vi "optionsAcq_interferogramSmoothing.vi"(0 "reference":refnum<class "OSA200.lvclass">, 2 "smoothing":T1, 4 "readWrite":enum16{"read", "write"}(ring), 5 "error in (no error)":errorcluster, 6 "width":u16, 7 "ignore range violation (false)":bool, 8 "nrOfPasses":u16) -> (10 "nrOfPasses out":u16, 12 "width out":u16, 14 "duplicate reference":refnum<class "OSA200.lvclass">, 15 "status":string, 16 "smoothing out":T1, 19 "error out":errorcluster)   [LabVIEW 2010, in "OSA200.lvclass"]
uses:
  OSA200.lvclass
  _misc/Thorlabs_FTS_misc.llb/interferogram_smoothing.ctl
  OSA.lvclass
  OSA20X_misc.lvlib
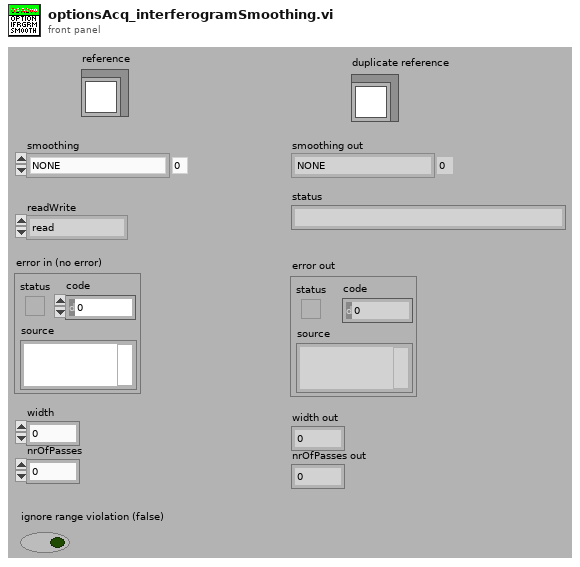
[diagram p1: front panel]
types:
  T1 = typedef "OSA20X_misc.lvlib/interferogram_smoothing.ctl" = enum16{"NONE", "BINOMIAL", "SAVITSKY_GOLAY", "FOURIER", "MOVING_AVERAGE", "GAUSSIAN"}
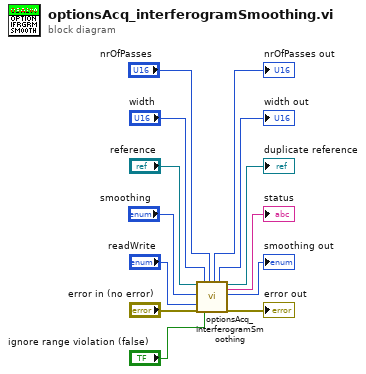
[diagram p0: block diagram]
diagram:
  n1 = call-parent "optionsAcq_interferogramSmoothing.vi"("reference"="reference", "smoothing"="smoothing", "readWrite"="readWrite", "error in (no error)"="error in (no error)", "width"="width", "ignore range violation (false)"="ignore range violation (false)", "nrOfPasses"="nrOfPasses") -> ("nrOfPasses out"=→"nrOfPasses out":u16, "width out"=→"width out":u16, "duplicate reference"=→"duplicate reference":refnum<class "OSA200.lvclass">, "status"=→"status":string, "smoothing out"=→"smoothing out":T1, "error out"=→"error out":errorcluster)  [unwired: 7 in]
